vi "Compass Page.vi"() -> ()   [LabVIEW 2020, in "2D Compass.lvclass"]
uses:
  <vilib>/Math Plots/2D Math Plots/2D Compass/2D Compass/2D Compass.lvclass
  <vilib>/Math Plots/2D Math Plots/2D Plot/Action String/2DMathPlot Ctrl Act Queue.ctl
  <vilib>/Math Plots/2D Math Plots/2D Plot/Action String/2DMathPlot Ctrl Act Cluster.ctl
  <vilib>/Math Plots/2D Math Plots/2D Plot/Action String/2DMathPlot State Class.ctl
  <vilib>/Math Plots/2D Math Plots/2D Compass/2D Compass/Typedef/2D Compass Property Cluster.ctl
  <vilib>/Math Plots/2D Math Plots/2D Plot/2D Plot/Typedef/Plot Property Array.ctl
  <vilib>/Math Plots/2D Math Plots/2D Plot/2D Plot/Typedef/Plot Property.ctl
  <vilib>/Math Plots/2D Math Plots/2D Compass/2D Compass/Typedef/2D Compass Property Array.ctl
  <vilib>/Math Plots/2D Math Plots/2D Compass/2D Compass/Typedef/2D Compass Property.ctl
  <vilib>/Math Plots/2D Math Plots/2D Plot/2D Plot/Typedef/Dialog State.ctl
  <vilib>/Math Plots/2D Math Plots/2D Plot/2D Plot/Typedef/Temp Graph State.ctl
  <vilib>/Math Plots/2D Math Plots/2D Plot/2D Plot/Typedef/Temp Graph Property Action.ctl
  <vilib>/Math Plots/2D Math Plots/2D Plot/2D Plot/2D Plot.lvclass
panel:
  in  "Line Color":u32(colorbox) caption="Color"
  out "Compass Property Out":T1={"Plot Property Array"=[{"Bar Plot Style"=0, "DigitalLineStyle"=1, "TransitionLocation"=2, "Transition Type"=0, "Fill To"=-1, "Fill/Pt. Color"=16448250, "Label Style"=3, "Line Style"=0, "Line Width"=0, "Plot Color"=16448250, "Plot Interpolation"=0, "Plot Name"="Plot 0", "Point Style"=1, "Visible?"=TRUE, "XScaleIdx"=0, "YScaleIdx"=0}, {"Bar Plot Style"=0, "DigitalLineStyle"=1, "TransitionLocation"=2, "Transition Type"=0, "Fill To"=-1, "Fill/Pt. Color"=16448250, "Label Style"=3, "Line Style"=0, "Line Width"=0, "Plot Color"=16448250, "Plot Interpolation"=0, "Plot Name"="Plot 1", "Point Style"=1, "Visible?"=TRUE, "XScaleIdx"=0, "YScaleIdx"=0}], "2D Compass Array"=[{"Compass Size"=2.0}, {"Compass Size"=2.0}], "Scale Visibility"={"Phase Scale"=TRUE}}
  in  "Compass Property In":T1={"Plot Property Array"=[{"Bar Plot Style"=0, "DigitalLineStyle"=1, "TransitionLocation"=2, "Transition Type"=0, "Fill To"=-1, "Fill/Pt. Color"=16448250, "Label Style"=3, "Line Style"=0, "Line Width"=0, "Plot Color"=16448250, "Plot Interpolation"=0, "Plot Name"="Plot 0", "Point Style"=1, "Visible?"=TRUE, "XScaleIdx"=0, "YScaleIdx"=0}, {"Bar Plot Style"=0, "DigitalLineStyle"=1, "TransitionLocation"=2, "Transition Type"=0, "Fill To"=-1, "Fill/Pt. Color"=16448250, "Label Style"=3, "Line Style"=0, "Line Width"=0, "Plot Color"=16448250, "Plot Interpolation"=0, "Plot Name"="Plot 1", "Point Style"=1, "Visible?"=TRUE, "XScaleIdx"=0, "YScaleIdx"=0}], "2D Compass Array"=[{"Compass Size"=2.0}, {"Compass Size"=2.0}], "Scale Visibility"={"Phase Scale"=TRUE}}
  in  "Control Ref Queue":T6
  in  "Event Registration":refnum<event-registration>
  in  "Phase Scale Visible":bool caption="Show phase scale"
  in  "Arrow Size":dbl=0.001 caption="Size" min=0.001 step=1.0
  in  "Line Width":T7
  in  "Line Style":T8
  in  "Name":string
  in  "Active Plot":i32(ring) items=["Plot 0"]
  # "Line"
  # "Compass"
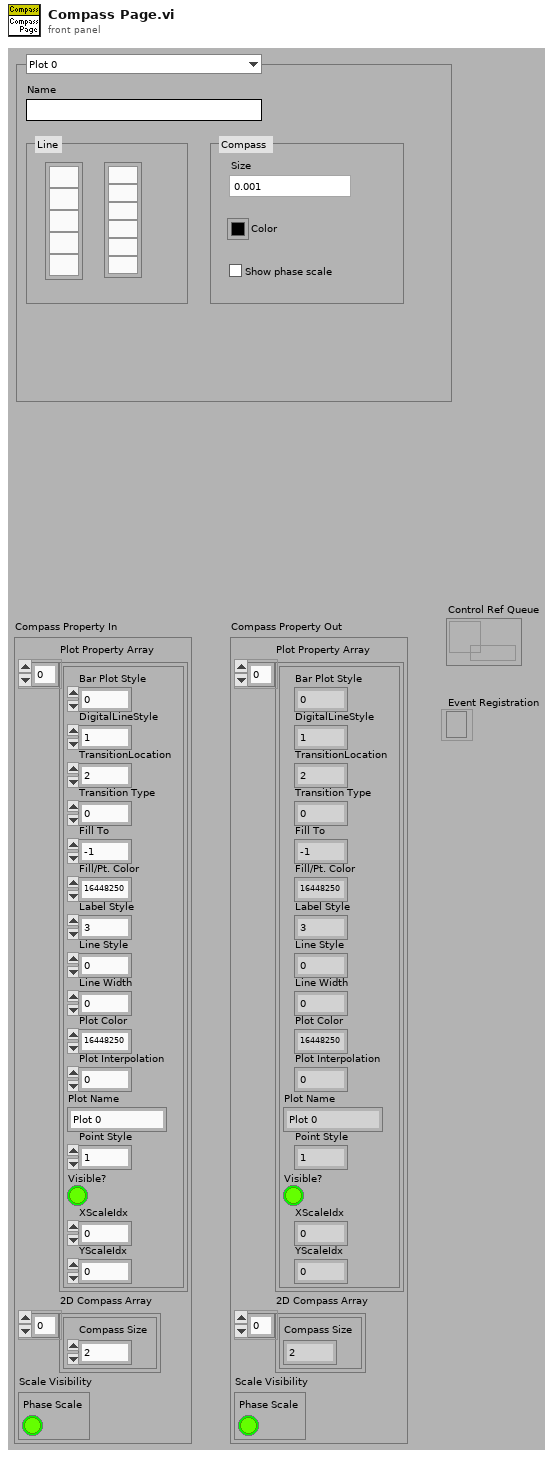
[diagram p1: front panel]
types:
  T1 = typedef "2D Compass.lvclass/2D Compass Property Cluster.ctl" = cluster{"Plot Property Array":T2, "2D Compass Array":T4, "Scale Visibility":cluster{"Phase Scale":bool}}
  T2 = typedef "2D Plot.lvclass/Plot Property Array.ctl" = T3[]
  T3 = typedef "2D Plot.lvclass/Plot Property.ctl" = cluster{"Bar Plot Style":u8, "DigitalLineStyle":u8, "TransitionLocation":u8, "Transition Type":u8, "Fill To":i16, "Fill/Pt. Color":u32, "Label Style":u8, "Line Style":u8, "Line Width":u8, "Plot Color":u32, "Plot Interpolation":u8, "Plot Name":string, "Point Style":u8, "Visible?":bool, "XScaleIdx":u32, "YScaleIdx":u32}
  T4 = typedef "2D Compass.lvclass/2D Compass Property Array.ctl" = T5[]
  T5 = typedef "2D Compass.lvclass/2D Compass Property.ctl" = cluster{"Compass Size":dbl}
  T6 = typedef "2DMathPlot Ctrl Act Queue.ctl" = refnum<queue>
  T7 = cluster{"OK Button 2":bool, "OK Button 3":bool, "OK Button 4":bool, "OK Button 5":bool, "OK Button 6":bool, "OK Button 7":bool}
  T8 = cluster{"OK Button":bool, "OK Button 2":bool, "OK Button 3":bool, "OK Button 4":bool, "OK Button 5":bool}
  T9 = typedef "2D Plot.lvclass/Dialog State.ctl" = enum16{"Initialize", "Read Property", "Write Property", "Idle", "Exit"}
  T10 = typedef "2DMathPlot Ctrl Act Cluster.ctl" = cluster{"Plot Area Ref":refnum<vi>, "Z Axis Ref":refnum<vi>, "Legend Ref":refnum<vi>, "XControl Ref":refnum<vi>, "Facade Ref":refnum<vi>, "Display State Change Class":T11}
  T11 = typedef "2DMathPlot State Class.ctl" = enum16{"Update All (Undo)", "Update General", "Update Appearance", "Update Format", "Update Scale", "Update Marker", "Update Cursor", "None"}
  T12 = typedef "2D Plot.lvclass/Temp Graph Property Action.ctl" = enum16{"Appearance Property", "Format Property", "Plots Property", "Scales Property"}
  T13 = typedef "2D Plot.lvclass/Temp Graph State.ctl" = enum16{"Create", "Update Graph", "Update Property Only", "Get Plot Name", "Get Axis Name", "Destory"}
  T14 = cluster{"Bool Array[0]":bool, "Bool Array[1]":bool, "Bool Array[2]":bool, "Bool Array[3]":bool, "Bool Array[4]":bool}
  T15 = cluster{"Bool Array[0]":bool, "Bool Array[1]":bool, "Bool Array[2]":bool, "Bool Array[3]":bool, "Bool Array[4]":bool, "Bool Array[5]":bool}
  T16 = typedef "LVPoint32TypeDef.ctl" = cluster{"Horizontal":i32, "Vertical":i32}
  T17 = typedef "LVRectTypeDef.ctl" = cluster{"left":i16, "top":i16, "right":i16, "bottom":i16}
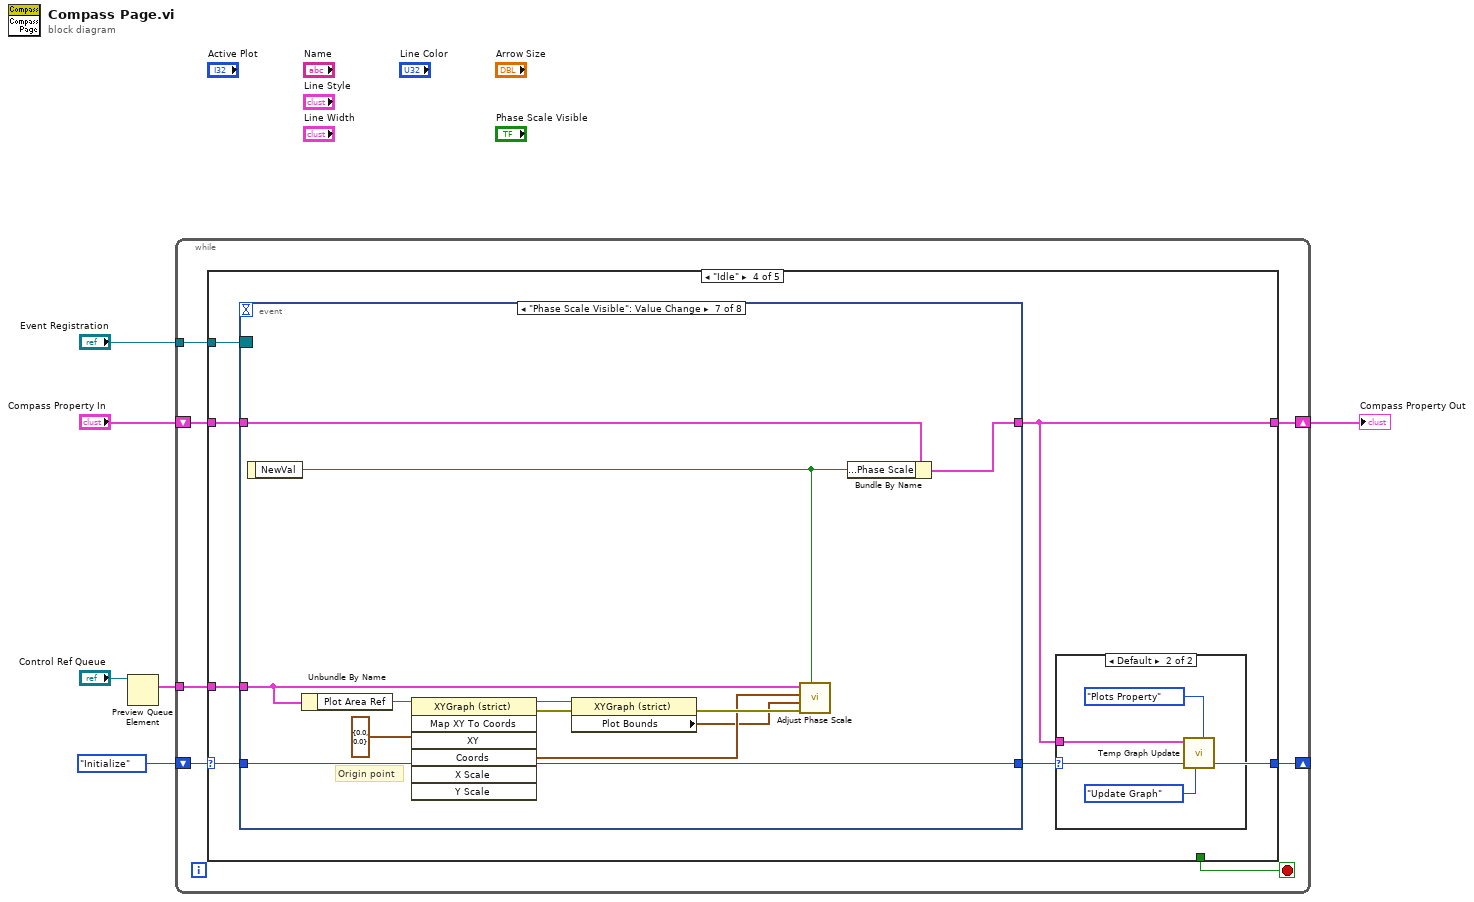
[diagram p0: block diagram]
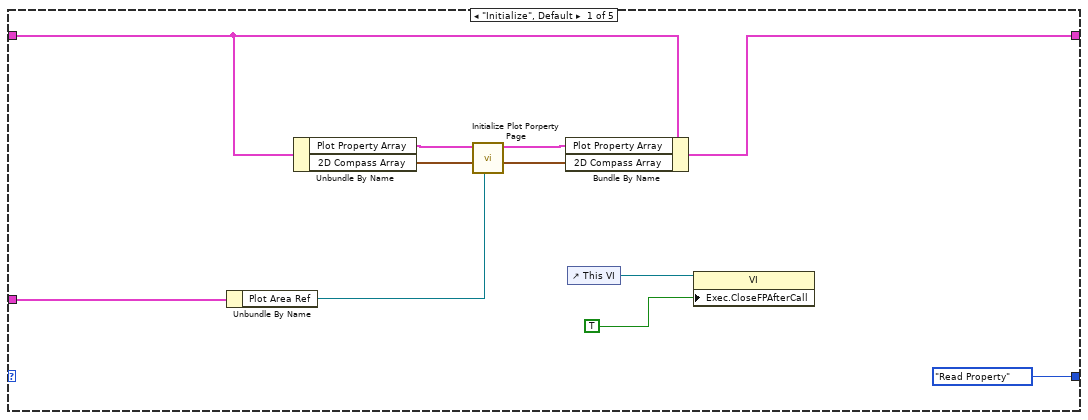
[diagram p2: hidden frame]
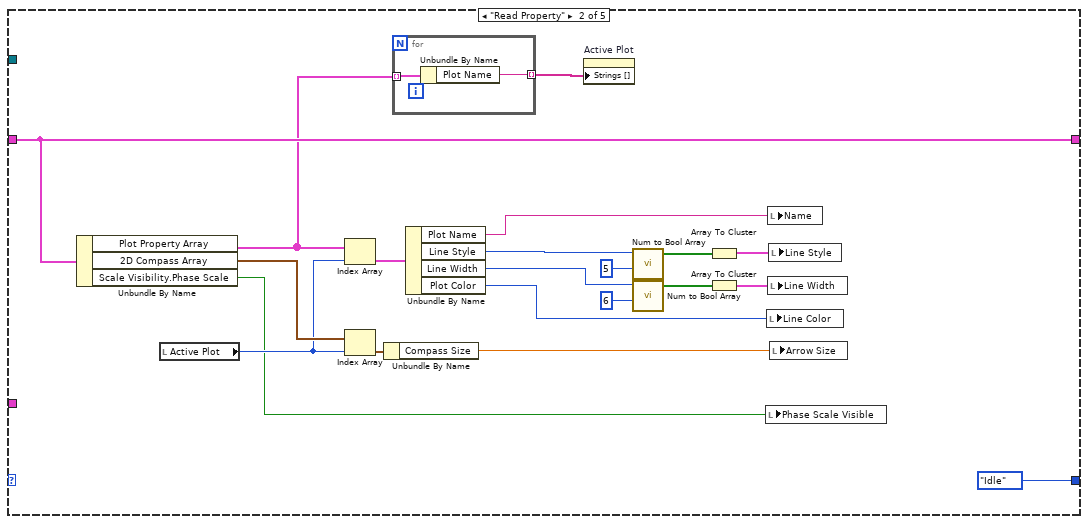
[diagram p3: hidden frame]
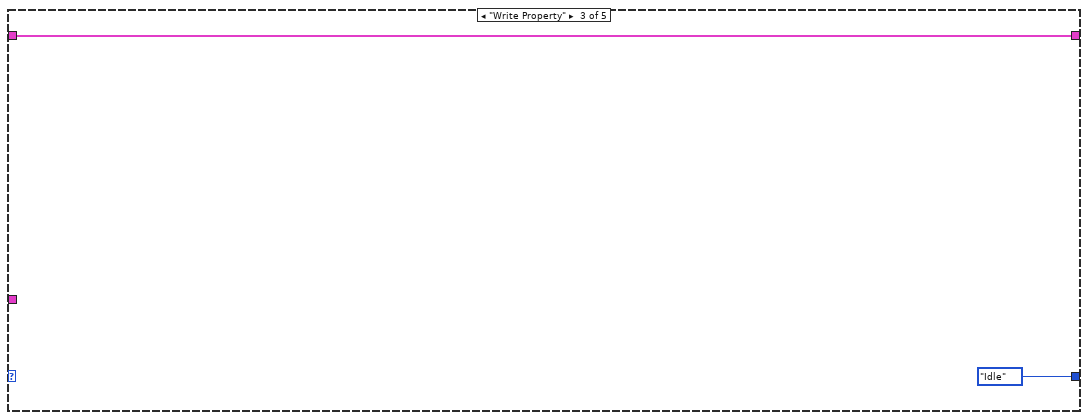
[diagram p4: hidden frame]
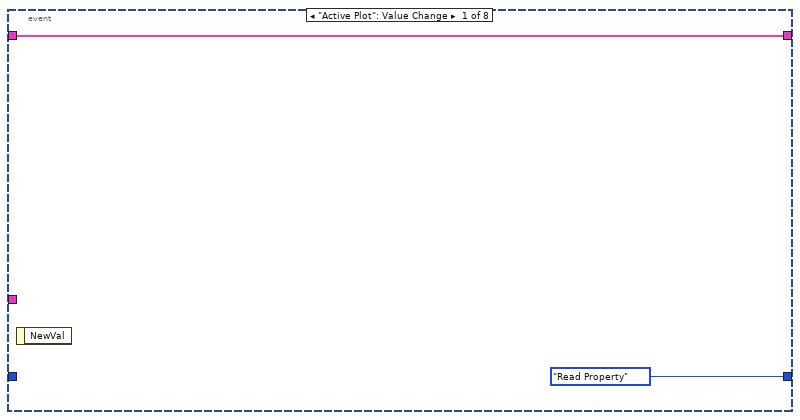
[diagram p6: hidden frame]
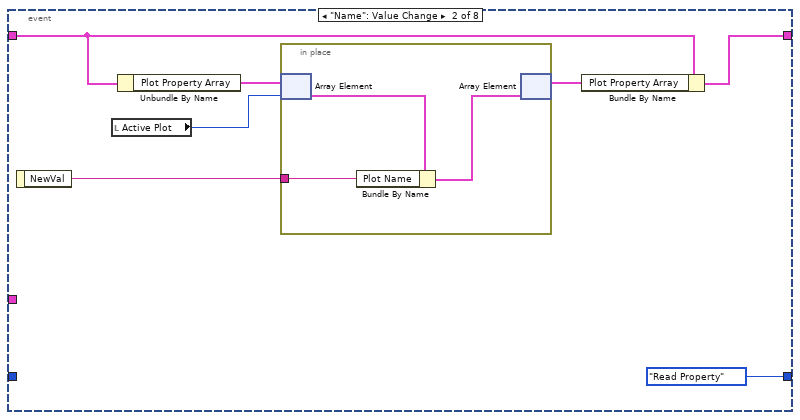
[diagram p7: hidden frame]
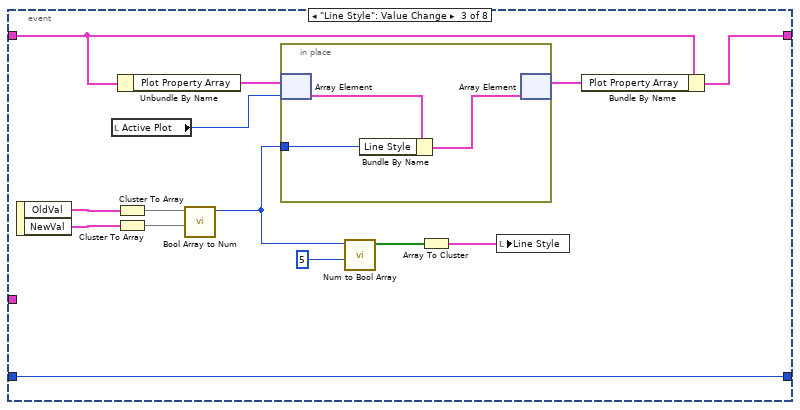
[diagram p8: hidden frame]
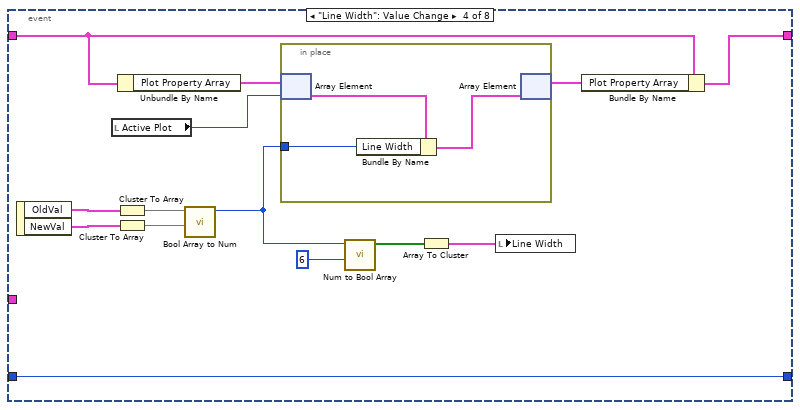
[diagram p9: hidden frame]
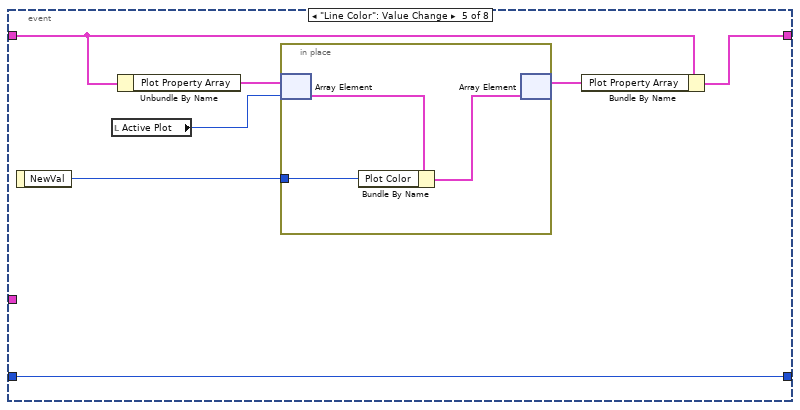
[diagram p10: hidden frame]
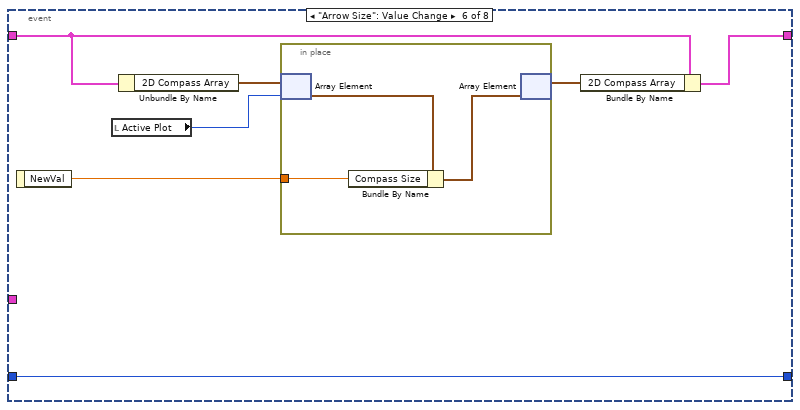
[diagram p11: hidden frame]
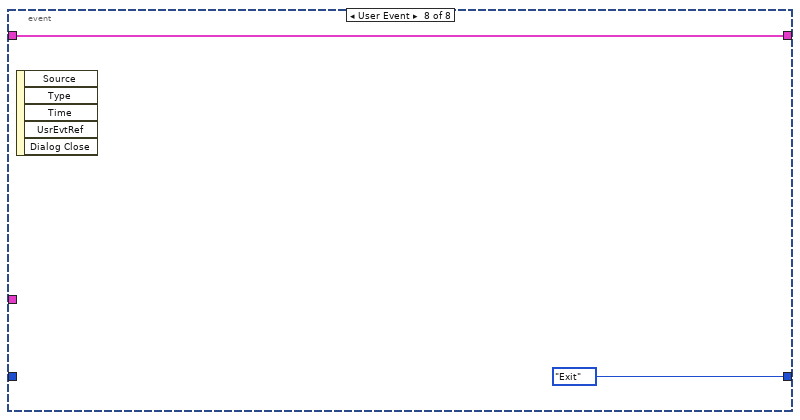
[diagram p12: hidden frame]
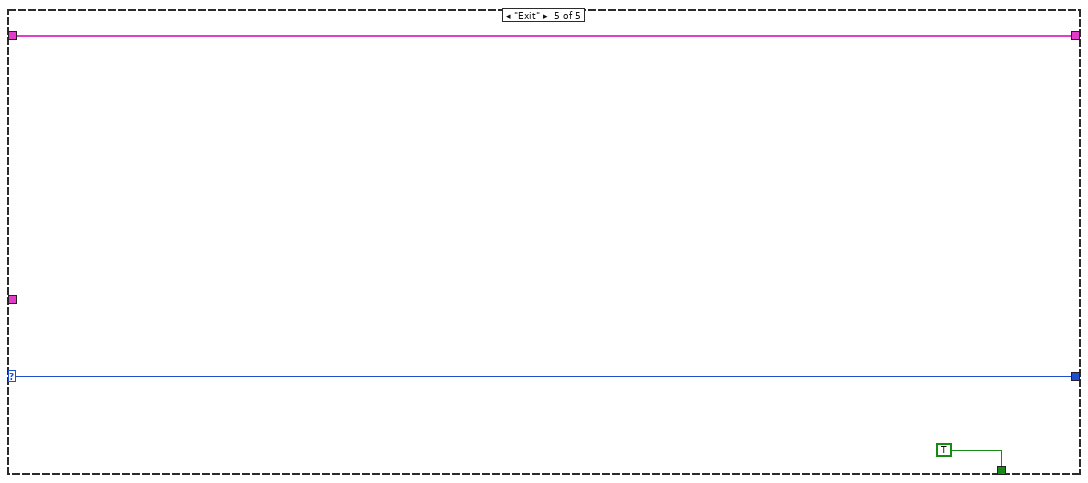
[diagram p13: hidden frame]
diagram:
  n1 = Preview Queue Element(queue="Control Ref Queue") -> (element=w1:T10)  [unwired: 1 in, 4 out]
  n2 = while {
    tunnel: "Event Registration" -> [w12]
    shift-right: [w9] -> _
    shift-left: Dialog_State."Initialize" ("Enum") -> [w13]
    shift-right: [w10] -> w2
    shift-left: "Compass Property In" -> [w11]
    tunnel: w1 -> [w7]
    stop <- w8 stop-if-true
    n3 = case shown="\"Idle\"" w13 {
      selector: w13 -> [_ _ _ w52 w140]
      tunnel: w12 -> [_ _ _ w54 _]
      tunnel: w11 -> [w21 w40 w47 w53 w138]
      tunnel: [w20 w40 w47 w51 w138] -> w10
      tunnel: [Dialog_State."Read Property" ("Enum") Dialog_State."Idle" ("Enum") Dialog_State."Idle" ("Enum") w50 w140] -> w9
      tunnel: [_ _ _ _ TRUE] -> w8
      tunnel: w7 -> [w15 _ _ w49 _]
      frame "Initialize", Default {
        n4 = Unbundle By Name(w15) -> ("Plot Area Ref"=w14:refnum<vi>)
        n5 = Unbundle By Name(w21) -> ("Plot Property Array"=w19:T2, "2D Compass Array"=w17:T4)
        n6 = call <vilib>:"Initialize Plot Porperty Page.vi"("Plot Area Ref"=w14, "2D Compass Array In"=w17, "Plot Property Array In"=w19) -> ("2D Compass Array Out"=w16:T4, "Plot Property Array Out"=w18:T2)  [unwired: 2 in, 5 out]
        n7 = Bundle By Name(cluster=w21, "Plot Property Array"=w18, "2D Compass Array"=w16) -> (w20:T1)
        n8 = control-ref of="This VI"() -> (w23:refnum<vi>)
        n9 = property class="VI"(reference=w23, "Exec.CloseFPAfterCall"=TRUE ("Execution:Close After Call")) -> ()  [unwired: 1 in, 2 out]
      }
      frame "Read Property" {
        n10 = Unbundle By Name(w40) -> ("Plot Property Array"=w26:T2, "2D Compass Array"=w44:T4, "Scale Visibility.Phase Scale"=w38:bool)
        n11 = local read "Active Plot"() -> (w43:i32)
        n12 = Index Array(array=w26, index=w43) -> (element=w42:T3)
        n13 = Index Array(array=w44, index=w43) -> (element=w41:T5)
        n14 = Unbundle By Name(w41) -> ("Compass Size"=w39:dbl)
        n15 = for {
          tunnel: w26 -> [w46] mode=indexing
          tunnel: [w45] -> w25 mode=indexing
          n16 = Unbundle By Name(w46) -> ("Plot Name"=w45:string)
        }
        n17 = Unbundle By Name(w42) -> ("Plot Name"=w37:string, "Line Style"=w36:u8, "Line Width"=w29:u8, "Plot Color"=w28:u32)
        n18 = property on="Active Plot" class="Ring (strict)"("Strings []"=w25) -> ()  [unwired: 2 in, 2 out]
        n19 = call <vilib>:"Num to Bool Array.vi"("Array Size"=5, "Value"=w36) -> ("Bool Array"=w34:bool[])  [unwired: 9 out]
        n20 = call <vilib>:"Num to Bool Array.vi"("Array Size"=6, "Value"=w29) -> ("Bool Array"=w32:bool[])  [unwired: 9 out]
        n21 = Array To Cluster(array=w34) -> (cluster=w33:T14)
        n22 = Array To Cluster(array=w32) -> (cluster=w30:T15)
        n23 = local write "Phase Scale Visible"(w38) -> ()
        n24 = local write "Line Color"(w28) -> ()
        n25 = local write "Name"(w37) -> ()
        n26 = local write "Line Width"(w30) -> ()
        n27 = local write "Line Style"(w33) -> ()
        n28 = local write "Arrow Size"(w39) -> ()
      }
      frame "Write Property" {
      }
      frame "Idle" {
        n29 = event shown="[6] \"Phase Scale Visible\": Value Change" {
          selector: w54 -> [_ _ _ _ _ _ _ _]
          dyn-events: _ -> [_ _ _ _ _ _ _ _]
          timeout: _ -> [_ _ _ _ _ _ _ _]
          tunnel: w53 -> [w59 w66 w83 w100 w110 w120 w135 w136]
          tunnel: [w59 w65 w82 w99 w109 w119 w134 w136] -> w51
          tunnel: [Dialog_State."Read Property" ("Enum") Dialog_State."Read Property" ("Enum") w70 w87 w105 w115 w133 Dialog_State."Exit" ("Enum")] -> w50
          tunnel: w52 -> [_ _ w70 w87 w105 w115 w133 _]
          tunnel: w49 -> [_ _ _ _ _ _ w126 _]
          event "Active Plot": Value Change {
            n30 = event-data() -> ()  [unwired: 2 out]
          }
          event "Name": Value Change {
            n31 = event-data() -> ("NewVal"=w61:string)  [unwired: 1 out]
            n32 = local read "Active Plot"() -> (w63:i32)
            n33 = Unbundle By Name(w66) -> ("Plot Property Array"=w64:T2)
            n34 = in-place {
              in-place-border: w61 -> [w67]
              n35 = in-place-array #1(w64, w63) -> (w69:T3)
              n36 = Bundle By Name(cluster=w69, "Plot Name"=w67) -> (w68:T3)
              n37 = in-place-array #1(w68) -> (w62:T2)  [unwired: 1 out]
            }
            n38 = Bundle By Name(cluster=w66, "Plot Property Array"=w62) -> (w65:T1)
          }
          event "Line Style": Value Change {
            n39 = event-data() -> ("OldVal"=w74:T8, "NewVal"=w73:T8)  [unwired: 1 out]
            n40 = local read "Active Plot"() -> (w80:i32)
            n41 = Cluster To Array(cluster=w74) -> (array=w76:bool[])
            n42 = Cluster To Array(cluster=w73) -> (array=w75:bool[])
            n43 = Unbundle By Name(w83) -> ("Plot Property Array"=w81:T2)
            n44 = call <vilib>:"Bool Array to Num.vi"("New Bool Array"=w75, "Old Bool Array"=w76) -> ("Value"=w71:u8)  [unwired: 9 out]
            n45 = in-place {
              in-place-border: w71 -> [w84]
              n46 = in-place-array #2(w81, w80) -> (w86:T3)
              n47 = Bundle By Name(cluster=w86, "Line Style"=w84) -> (w85:T3)
              n48 = in-place-array #2(w85) -> (w79:T2)  [unwired: 1 out]
            }
            n49 = call <vilib>:"Num to Bool Array.vi"("Array Size"=5, "Value"=w71) -> ("Bool Array"=w78:bool[])  [unwired: 9 out]
            n50 = Array To Cluster(array=w78) -> (cluster=w72:T14)
            n51 = local write "Line Style"(w72) -> ()
            n52 = Bundle By Name(cluster=w83, "Plot Property Array"=w79) -> (w82:T1)
          }
          event "Line Width": Value Change {
            n53 = event-data() -> ("OldVal"=w91:T7, "NewVal"=w90:T7)  [unwired: 1 out]
            n54 = local read "Active Plot"() -> (w97:i32)
            n55 = Cluster To Array(cluster=w91) -> (array=w93:bool[])
            n56 = Cluster To Array(cluster=w90) -> (array=w92:bool[])
            n57 = Unbundle By Name(w100) -> ("Plot Property Array"=w98:T2)
            n58 = call <vilib>:"Bool Array to Num.vi"("New Bool Array"=w92, "Old Bool Array"=w93) -> ("Value"=w88:u8)  [unwired: 9 out]
            n59 = in-place {
              in-place-border: w88 -> [w101]
              n60 = in-place-array #3(w98, w97) -> (w103:T3)
              n61 = Bundle By Name(cluster=w103, "Line Width"=w101) -> (w102:T3)
              n62 = in-place-array #3(w102) -> (w96:T2)  [unwired: 1 out]
            }
            n63 = call <vilib>:"Num to Bool Array.vi"("Array Size"=6, "Value"=w88) -> ("Bool Array"=w95:bool[])  [unwired: 9 out]
            n64 = Array To Cluster(array=w95) -> (cluster=w89:T15)
            n65 = local write "Line Width"(w89) -> ()
            n66 = Bundle By Name(cluster=w100, "Plot Property Array"=w96) -> (w99:T1)
          }
          event "Line Color": Value Change {
            n67 = event-data() -> ("NewVal"=w104:u32)  [unwired: 1 out]
            n68 = local read "Active Plot"() -> (w107:i32)
            n69 = Unbundle By Name(w110) -> ("Plot Property Array"=w108:T2)
            n70 = in-place {
              in-place-border: w104 -> [w111]
              n71 = in-place-array #4(w108, w107) -> (w113:T3)
              n72 = Bundle By Name(cluster=w113, "Plot Color"=w111) -> (w112:T3)
              n73 = in-place-array #4(w112) -> (w106:T2)  [unwired: 1 out]
            }
            n74 = Bundle By Name(cluster=w110, "Plot Property Array"=w106) -> (w109:T1)
          }
          event "Arrow Size": Value Change {
            n75 = event-data() -> ("NewVal"=w114:dbl)  [unwired: 1 out]
            n76 = local read "Active Plot"() -> (w117:i32)
            n77 = Unbundle By Name(w120) -> ("2D Compass Array"=w118:T4)
            n78 = in-place {
              in-place-border: w114 -> [w121]
              n79 = in-place-array #5(w118, w117) -> (w123:T5)
              n80 = Bundle By Name(cluster=w123, "Compass Size"=w121) -> (w122:T5)
              n81 = in-place-array #5(w122) -> (w116:T4)  [unwired: 1 out]
            }
            n82 = Bundle By Name(cluster=w120, "2D Compass Array"=w116) -> (w119:T1)
          }
          event "Phase Scale Visible": Value Change {
            # "Origin point"
            n83 = event-data() -> ("NewVal"=w127:bool)  [unwired: 1 out]
            n84 = Unbundle By Name(w126) -> ("Plot Area Ref"=w125:refnum<vi>)
            n85 = invoke on="Invoke Node" class="XYGraph (strict)" method="Map XY To Coords"(reference=w125, "XY"=cluster{"X":dbl, "Y":dbl} {"X"=0.0, "Y"=0.0}) -> (reference out=w128:refnum<vi>, error out=w130:errorcluster, "Coords"=w131:T16)  [unwired: 5 in, 4 out]
            n86 = property class="XYGraph (strict)"(reference=w128, error in=w130) -> (error out=w132:errorcluster, "Plot Bounds"=w124:T17)  [unwired: 1 out]
            n87 = call <vilib>:"Adjust Phase Scale.vi"("Show Scale?"=w127, "error in (no error)"=w132, "Plot Area Bounds"=w124, "Origin Coords"=w131, "Control Ref Cluster"=w126) -> ()  [unwired: 7 out]
            n88 = Bundle By Name(cluster=w135, "Scale Visibility.Phase Scale"=w127) -> (w134:T1)
          }
          event User Event {
            n89 = event-data() -> ()  [unwired: 6 out]
          }
        }
        n90 = case shown="Default" w50 {
          tunnel: w51 -> [_ w55]
          frame "Exit" {
          }
          frame Default {
            n91 = call <vilib>:"Temp Graph Update.vi"("Property Name"=Temp_Graph_Property_Action."Plots Property", "State"=Temp_Graph_State."Update Graph", "Property In"=w55) -> ()  [unwired: 2 in, 7 out]
          }
        }
      }
      frame "Exit" {
      }
    }
  }
  "Compass Property Out" <- w2
